vi "BuildMsg (Core).vi"(8 "error in (no error)":errorcluster, 9 "ProgressBarCluster":T1, 10 "Msg to be build":string, 11 "CS++Actor in":refnum<class "CS++Actor.lvclass">) -> (0 "error out":errorcluster, 2 "ActiveMessageClass":refnum<vi>, 3 "CS++Actor out":refnum<class "CS++Actor.lvclass">)   [LabVIEW 2014, in "CS++Actor.lvlib" / "CS++Actor.lvclass"]
doc: "Core of the Build Msg command."
uses:
  CS++Actor.lvclass
  CS++Actor.lvclass/CS++Actor.ctl
  CSPP_MessageMaker_Utilities/CS++MessagemakerUtilities.lvlib
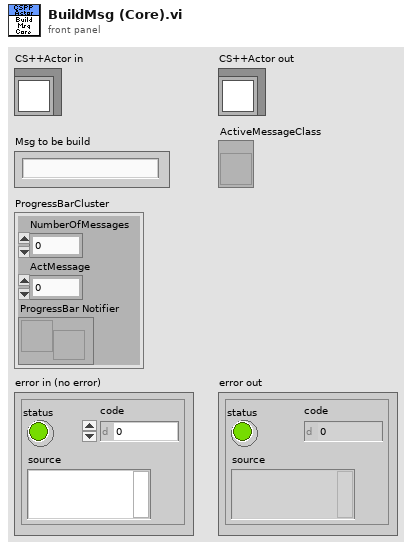
[diagram p1: front panel]
types:
  T1 = cluster{"NumberOfMessages":u16, "ActMessage":u16, "ProgressBar Notifier":refnum<notifier>}
  T2 = cluster{"Actor":cluster{"In":i32, "Out":i32}, "Error":cluster{"In":i32, "Out":i32}, "Terminals":cluster{"Position":enum16{"Left", "Top", "Bottom", "Right"}, "Terminal":i32}[]}
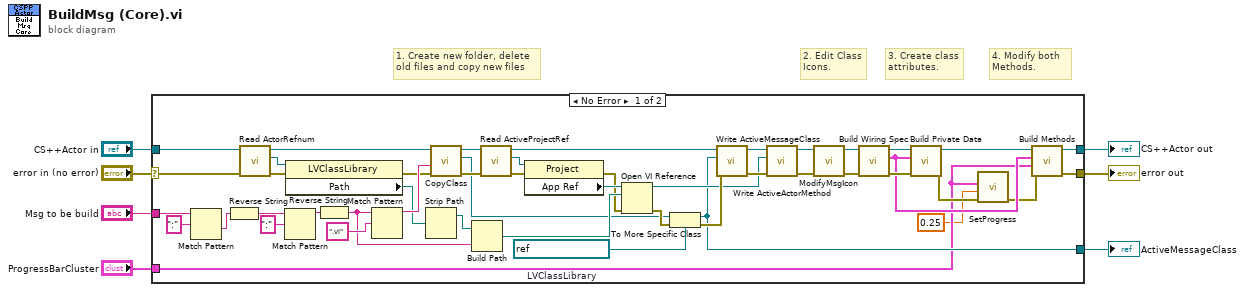
[diagram p0: block diagram]
diagram:
  # "2. Edit Class\nIcons."
  # "4. Modify both\nMethods."
  # "3. Create class\nattributes."
  # "1. Create new folder, delete\nold files and copy new files"
  n1 = case shown="No Error" "error in (no error)" {
    selector: "error in (no error)" -> [w33 w56]
    tunnel: [w12 w56] -> w6
    tunnel: [w13 w55] -> w4
    tunnel: "CS++Actor in" -> [w32 w55]
    tunnel: "Msg to be build" -> [w49 _]
    tunnel: [w19 _] -> w2
    tunnel: "ProgressBarCluster" -> [w15 _]
    frame No Error {
      w40 = refnum<vi> refnum  # LVClassLibrary
      n2 = Match Pattern(string=w49, regular expression=":") -> (after substring=w48:string)  [unwired: 1 in, 3 out]
      n3 = Reverse String(1:w48) -> (0:w54:string)
      n4 = call "Read ActorRefnum.vi"("error in (no error)"=w33, "CS++Actor in"=w32) -> ("error out"=w35:errorcluster, "ActorRefnum"=w34:refnum<vi>, "CS++Actor out"=w31:refnum<class "CS++Actor.lvclass">)  [unwired: 7 in]
      n5 = Match Pattern(string=w54, regular expression=":") -> (before substring=w52:string)  [unwired: 1 in, 3 out]
      n6 = property class="LVClassLibrary"(reference=w34, error in=w35) -> (error out=w30:errorcluster, "Path"=w29:path)  [unwired: 1 out]
      n7 = Reverse String(1:w52) -> (0:w47:string)
      n8 = Match Pattern(string=w47, regular expression=".vi") -> (before substring=w36:string)  [unwired: 1 in, 3 out]
      n9 = Strip Path(path=w29) -> (stripped path=w46:path)  [unwired: 1 out]
      n10 = call "CopyClass.vi"("error in (no error)"=w30, "Actor Method VI Name"=w36, "CS++Actor in"=w31) -> ("error out"=w38:errorcluster, "AddItemFromMemory"=w20:refnum<vi>, "CS++Actor out"=w37:refnum<class "CS++Actor.lvclass">)  [unwired: 5 in, 1 out]
      n11 = Build Path(base path=w46, name or relative path=w47) -> (appended path=w45:path)
      n12 = call "Read ActiveProjectRef.vi"("error in (no error)"=w38, "CS++Actor in"=w37) -> ("error out"=w42:errorcluster, "ActiveProjectRef"=w44:refnum<vi>, "CS++Actor out"=w28:refnum<class "CS++Actor.lvclass">)  [unwired: 7 in]
      n13 = property class="Project"(reference=w44, error in=w42) -> (error out=w41:errorcluster, "App Ref"=w43:refnum<vi>)  [unwired: 1 out]
      n14 = Open VI Reference(application reference (local)=w43, vi path=w45, error in (no error)=w41) -> (vi reference=w24:refnum<vi>, error out=w39:errorcluster)  [unwired: 3 in]
      n15 = To More Specific Class(target class=w40, reference=w20, error in=w39) -> (specific class reference=w19:refnum<vi>, error out=w27:errorcluster)
      n16 = call "Write ActiveMessageClass.vi"("error in (no error)"=w27, "ActiveMessageClass"=w19, "CS++Actor in"=w28) -> ("error out"=w26:errorcluster, "CS++Actor out"=w25:refnum<class "CS++Actor.lvclass">)  [unwired: 7 in]
      n17 = call "Write ActiveActorMethod.vi"("error in (no error)"=w26, "ActiveActorMethod"=w24, "CS++Actor in"=w25) -> ("error out"=w10:errorcluster, "CS++Actor out"=w11:refnum<class "CS++Actor.lvclass">)  [unwired: 7 in]
      n18 = call "ModifyMsgIcon.vi"("error in (no error)"=w10, "CS++Actor in"=w11) -> ("error out"=w9:errorcluster, "CS++Actor out"=w8:refnum<class "CS++Actor.lvclass">)  [unwired: 8 in]
      n19 = call "Build Wiring Spec.vi"("error in (no error)"=w9, "CS++Actor in"=w8) -> ("error out"=w22:errorcluster, "Wiring Spec"=w18:T2, "CS++Actor out"=w21:refnum<class "CS++Actor.lvclass">)  [unwired: 7 in]
      n20 = call "Build Private Data.vi"("error in (no error)"=w22, "Wiring Spec"=w18, "CS++Actor in"=w21) -> ("error out"=w17:errorcluster, "CS++Actor out"=w23:refnum<class "CS++Actor.lvclass">)  [unwired: 7 in]
      n21 = call "SetProgress.vi"("error in (no error)"=w17, "SubStep"=0.25, "ProgressBarCluster"=w15) -> ("error out"=w16:errorcluster)  [unwired: 8 in]
      n22 = call "Build Methods.vi"("error in (no error)"=w16, "ProgressBarCluster"=w15, "Wiring Spec"=w18, "CS++Actor in"=w23) -> ("error out"=w12:errorcluster, "CS++Actor out"=w13:refnum<class "CS++Actor.lvclass">)  [unwired: 6 in]
    }
    frame Error {
    }
  }
  "error out" <- w6
  "CS++Actor out" <- w4
  "ActiveMessageClass" <- w2
